vi "Set-Get_format_test.vi"() -> (0 "Test_passed":bool)   [LabVIEW 2014]
panel:
  out "Values_actualy_read":string[](array[string])=["-35", "\"adios\"", "true", "0.100000", "1.000000E+11", "1.500000E+17", "-2.130000", "1.500000E-5", "false"]
  in  "values to set":string[](array[string])=["-35", "adios", "true", "0.1", "100000000000", "1.5E17", "-2.13", "1.5e-5", "false"]
  in  "Expected values to read":string[](array[string])=["-35", "\"adios\"", "true", "0.100000", "1.000000E+11", "1.500000E+17", "-2.130000", "1.500000E-5", "false"]
  in  "variables":string[](array[string])=["intin", "stringin", "booleanin", "doublein", "doublein", "doublein", "doublein", "doublein", "booleanin"]
  out "hidden3":errorcluster
  out "hidden":errorcluster
  in  "Experience ID1":string="TestOK"
  out "Test_OK":bool[](array[boolean])=[TRUE, FALSE, TRUE, TRUE, TRUE, TRUE, TRUE, TRUE, TRUE]
  # "read in SEQUENCE not in block as usual"
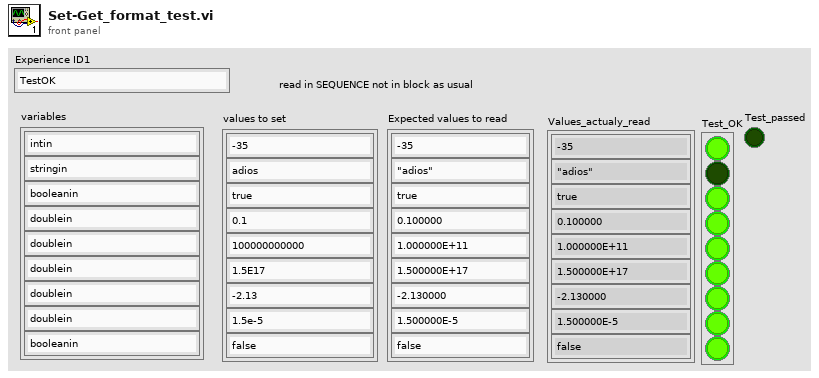
[diagram p1: front panel]
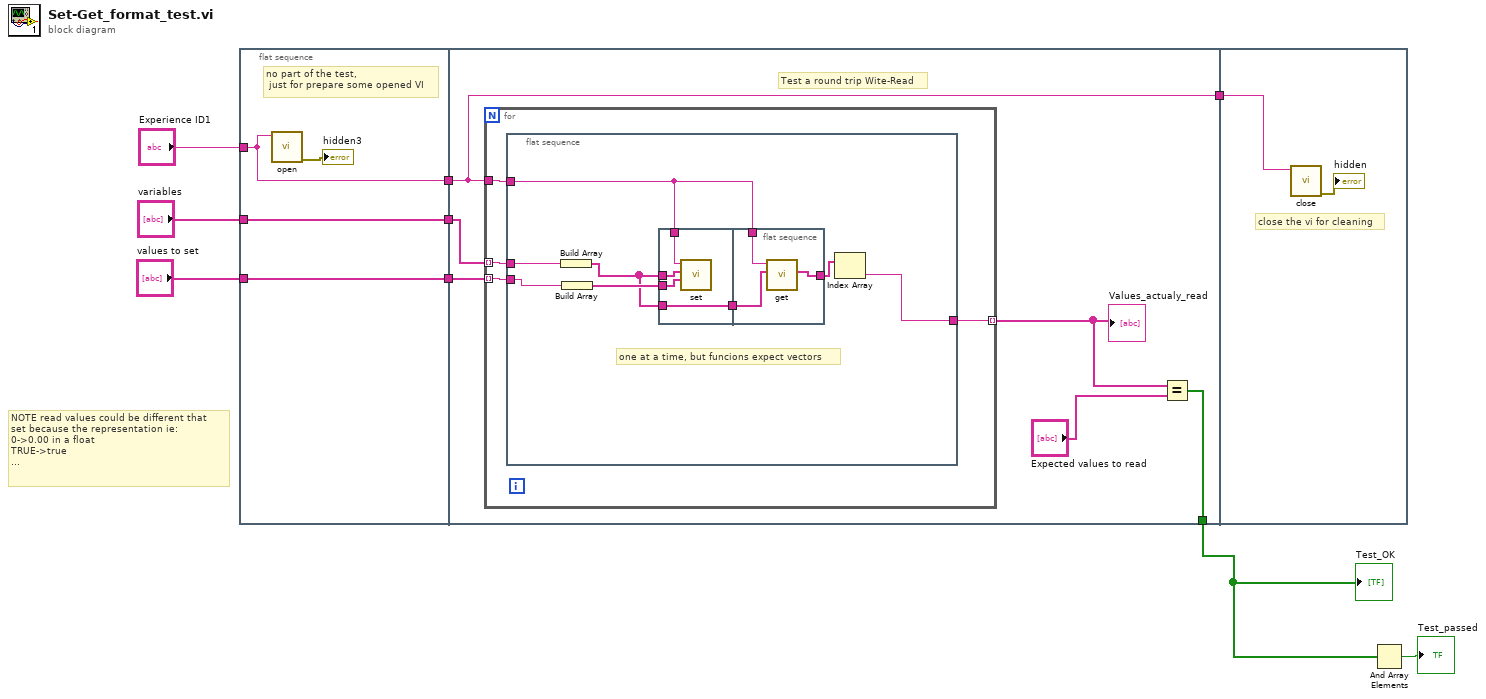
[diagram p0: block diagram]
diagram:
  # "NOTE read values could be different that \nset because the representation ie:\n0->0.00 in a float\nTRUE->true\n..."
  n1 = flat-sequence {
    tunnel: "Experience ID1" -> [w12]
    tunnel: [w12] -> w6
    tunnel: [w11] -> w5
    tunnel: "variables" -> [w11]
    tunnel: [w10] -> w4
    tunnel: "values to set" -> [w10]
    tunnel: w6 -> [w17]
    tunnel: w5 -> [w19]
    tunnel: w4 -> [w18]
    tunnel: [w17] -> w2
    tunnel: [w14] -> w1
    tunnel: w2 -> [w39]
    frame #0 {
      # "no part of the test,\n just for prepare some opened VI"
      n2 = call "open.vi"("Experience ID"=w12) -> ("error out"=→"hidden3":errorcluster)  [unwired: 8 in, 2 out]
    }
    frame #1 {
      # "Test a round trip Wite-Read"
      n3 = for {
        tunnel: w17 -> [w23]
        tunnel: w19 -> [w22] mode=indexing
        tunnel: w18 -> [w21] mode=indexing
        tunnel: [w20] -> w16 mode=indexing
        n4 = flat-sequence {
          tunnel: w23 -> [w30]
          tunnel: w22 -> [w31]
          tunnel: w21 -> [w28]
          tunnel: [w24] -> w20
          frame #0 {
            # "one at a time, but funcions expect vectors"
            n5 = Build Array(w31) -> (w26:string[])
            n6 = Build Array(w28) -> (w29:string[])
            n7 = flat-sequence {
              tunnel: w30 -> [w35]
              tunnel: w26 -> [w34]
              tunnel: w29 -> [w33]
              tunnel: [w32] -> w27
              tunnel: w26 -> [w32]
              tunnel: w30 -> [w38]
              tunnel: w27 -> [w37]
              tunnel: [w36] -> w25
              frame #0 {
                n8 = call "set.vi"("values"=w33, "variables"=w34, "Experience ID"=w35) -> ()  [unwired: 8 in, 1 out]
              }
              frame #1 {
                n9 = call "get.vi"("variables"=w37, "Experience ID"=w38) -> ("values"=w36:string[])  [unwired: 7 in, 2 out]
              }
            }
            n10 = Index Array(array=w25) -> (element=w24:string)  [unwired: 1 in]
          }
        }
      }
      "Values_actualy_read" <- w16
      n11 = Equal?(x=w16, y="Expected values to read") -> (x = y?=w14:bool[])
    }
    frame #2 {
      # "close the vi for cleaning"
      n12 = call "close.vi"("Experience ID"=w39) -> ("error out"=→"hidden":errorcluster)  [unwired: 10 in]
    }
  }
  n13 = And Array Elements(Boolean array=w1) -> (logical AND=→"Test_passed":bool)
  "Test_OK" <- w1
